vi "init.vi"(8 "error in":errorcluster, 10 "TBM module configuration in":refnum<class "TBM module configuration.lvclass">, 11 "CVT runtime in":refnum<class "CVT runtime.lvclass">) -> (0 "error out":errorcluster, 1 "data allocations":T1, 2 "execution settings":T4, 3 "CVT runtime out":refnum<class "CVT runtime.lvclass">)   [LabVIEW 2013, in "CVT runtime.lvclass"]
doc: "Provides an interface for initializing a module at runtime. While this interface performs no operations, a child should provide an override which may open any necessary references or sessions, allocate necessary memory, and perform any final configuration validataion before providing the full configuration <b>execution data</b> to the calling process."
uses:
  CVT runtime.lvclass
  <vilib>/NI/Tag Bus Module Framework/module configuration/TBM module configuration.lvclass
  <vilib>/NI/Tag Bus Module Framework/runtime/execution settings.ctl
  <vilib>/NI/Tag Bus Module Framework/channel/data tables.ctl
  <vilib>/NI/Tag Bus/dictionary/data dictionary.lvclass
  <vilib>/NI/Tag Bus/dictionary table pair.ctl
  <vilib>/NI/Tag Bus/table/data table.ctl
  configuration/CVT configuration.lvclass
  CVT runtime.lvclass/CVT runtime.ctl
  <vilib>/NI/Tag Bus Module Framework/channel/TBM channel.lvclass
  <vilib>/NI/Tag Bus Module Framework/runtime/TBM module execution interface.lvclass
  <vilib>/NI/Tag Bus/tag bus.lvlib
  <vilib>/NI/Tag Bus/table/data table.lvlib
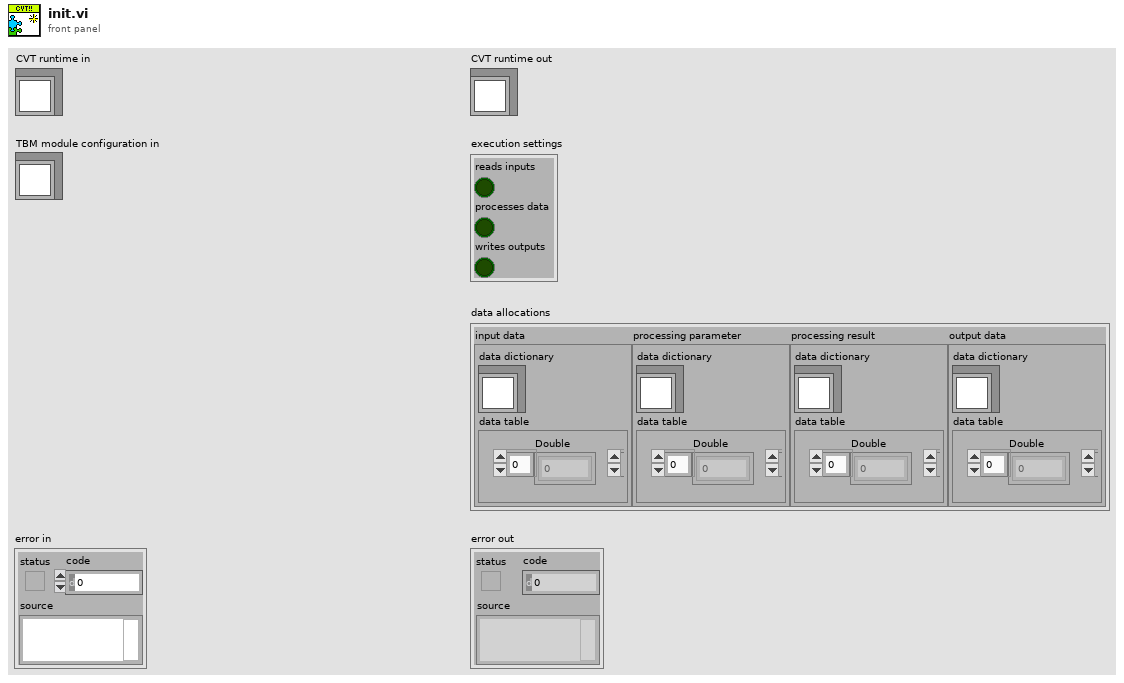
[diagram p1: front panel]
types:
  T1 = typedef "TBM channel.lvclass/data tables.ctl" = cluster{"input data":T2, "processing parameter":T2, "processing result":T2, "output data":T2}
  T2 = typedef "tag bus.lvlib/dictionary table pair.ctl" = cluster{"data dictionary":refnum<class "data dictionary.lvclass">, "data table":T3}
  T3 = typedef "tag bus.lvlib/data table.lvlib/data table.ctl" = cluster{"Double":dbl[], "Single":sgl[], "I64":i64[], "I32":i32[], "I16":i16[], "I8":i8[], "U64":u64[], "U32":u32[], "U16":u16[], "U8":u8[], "Boolean":bool[], "String":string[], "Array of Double":cluster{"DBL Array":dbl[]}[], "Array of Single":cluster{"SGL Array":sgl[]}[], "Array of I64":cluster{"I64 Array":i64[]}[], "Array of I32":cluster{"I32 Array":i32[]}[], "Array of I16":cluster{"I16 Array":i16[]}[], "Array of I8":cluster{"I8 Array":i8[]}[], "Array of U64":cluster{"U64 Array":u64[]}[], "Array of U32":cluster{"U32 Array":u32[]}[], "Array of U16":cluster{"U16 Array":u16[]}[], "Array of U8":cluster{"U8 Array":u8[]}[], "Array of Boolean":cluster{"Boolean Array":bool[]}[], "Array of String":cluster{"String Array":string[]}[]}
  T4 = typedef "TBM module execution interface.lvclass/execution settings.ctl" = cluster{"reads inputs":bool, "processes data":bool, "writes outputs":bool}
  T5 = typedef "Current Value Table.lvlib/Typed Index Set.ctl" = cluster{"Data Type":T6, "Indices":i32[]}
  T6 = typedef "Current Value Table.lvlib/Data Types.ctl" = enum16{"Double", "Single", "I64", "I32", "I16", "I8", "U64", "U32", "U16", "U8", "String", "Boolean", "Array of U8", "Array of U16", "Array of U32", "Array of U64", "Array of I64", "Array of I32", "Array of I16", "Array of I8", "Array of Double", "Array of Single", "Array of Boolean", "Array of String"}
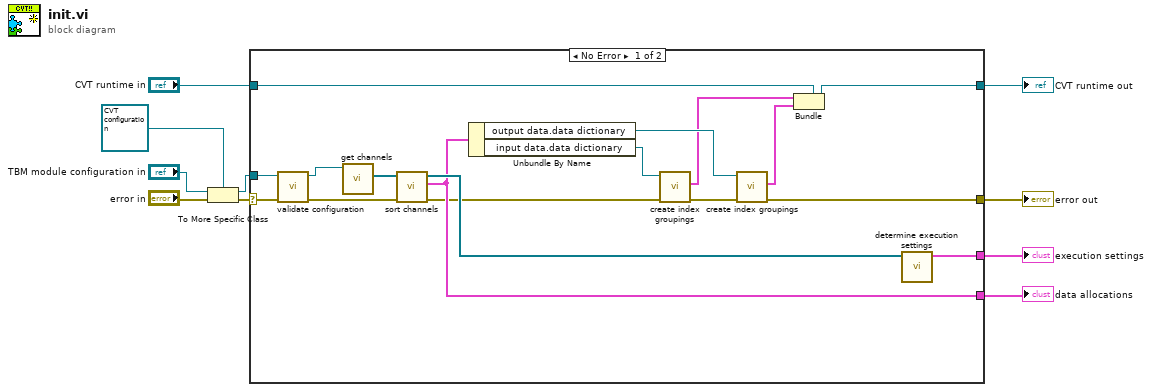
[diagram p0: block diagram]
diagram:
  n1 = To More Specific Class(target class=refnum<class "CVT configuration.lvclass"> refnum ("CVT configuration"), reference="TBM module configuration in", error in="error in") -> (specific class reference=w9:refnum<class "CVT configuration.lvclass">, error out=w10:errorcluster)
  n2 = case shown="No Error" w10 {
    selector: w10 -> [w23 w28]
    tunnel: w9 -> [w11 _]
    tunnel: "CVT runtime in" -> [w27 w29]
    tunnel: [w20 w29] -> w5
    tunnel: [w16 w28] -> w4
    tunnel: [w19 _] -> w2
    tunnel: [w26 _] -> w3
    frame No Error {
      n3 = call-dynamic "validate configuration.vi"("error in"=w23, "CVT configuration in"=w11) -> ("error out"=w24:errorcluster, "CVT configuration out"=w22:refnum<class "CVT configuration.lvclass">)  [unwired: 8 in]
      n4 = call-dynamic "get channels.vi"("CVT configuration in"=w22) -> ("channels"=w21:refnum<class "TBM channel.lvclass">[])  [unwired: 9 in, 1 out]
      n5 = call <vilib>:"sort channels.vi"("error in"=w24, "channels in"=w21) -> ("error out"=w18:errorcluster, "data allocations"=w19:T1, "channels out"=w25:refnum<class "TBM channel.lvclass">[])  [unwired: 7 in]
      n6 = Unbundle By Name(w19) -> ("output data.data dictionary"=w15:refnum<class "data dictionary.lvclass">, "input data.data dictionary"=w14:refnum<class "data dictionary.lvclass">)
      n7 = call "create index groupings.vi"("error in"=w18, "data dictionary"=w14) -> ("error out"=w17:errorcluster, "indices"=w13:T5[])  [unwired: 8 in]
      n8 = call "create index groupings.vi"("error in"=w17, "data dictionary"=w15) -> ("error out"=w16:errorcluster, "indices"=w12:T5[])  [unwired: 8 in]
      n9 = Bundle(cluster=w27, w13, w12) -> (w20:refnum<class "CVT runtime.lvclass">)
      n10 = call <vilib>:"determine execution settings.vi"("channels"=w25) -> ("execution settings"=w26:T4)  [unwired: 10 in]
    }
    frame Error {
    }
  }
  "error out" <- w4
  "CVT runtime out" <- w5
  "execution settings" <- w3
  "data allocations" <- w2
